vi "Non-SD UI Ref.vi"(8 "error in (no error)":errorcluster, 11 "9402 in":refnum<class "9402.lvclass">) -> (0 "error out":errorcluster, 1 "Show SubPanel?":bool, 2 "VI Refnum":refnum<vi>, 3 "9402 out":refnum<class "9402.lvclass">)   [LabVIEW 2017, in "Modules.lvlib" / "9402.lvclass"]
uses:
  9402.lvclass
  9402_UI.vi
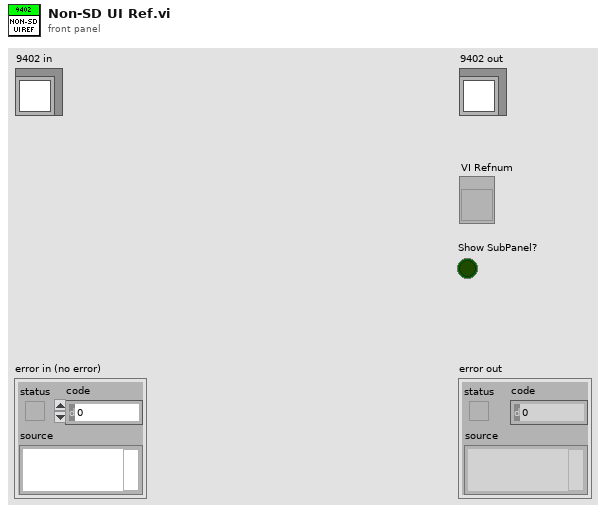
[diagram p1: front panel]
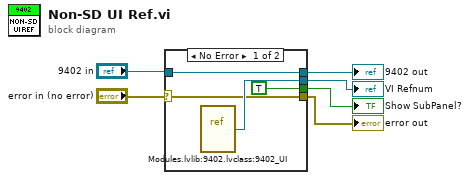
[diagram p0: block diagram]
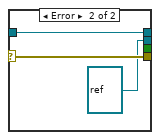
[diagram p2: hidden frame]
diagram:
  n1 = case shown="No Error" "error in (no error)" {
    selector: "error in (no error)" -> [w7 w13]
    tunnel: [w7 w13] -> w1
    tunnel: [w8 w12] -> w4
    tunnel: "9402 in" -> [w8 w12]
    tunnel: [w10 refnum<vi> refnum] -> w3
    tunnel: [TRUE _] -> w2
    frame No Error {
      n2 = vi-ref "Modules.lvlib:9402.lvclass:9402_UI.vi"() -> (w10:refnum<vi>)
    }
    frame Error {
    }
  }
  "error out" <- w1
  "9402 out" <- w4
  "VI Refnum" <- w3
  "Show SubPanel?" <- w2
